vi "Test Basic Forms.vi"() -> ()   [LabVIEW 2020]
uses:
  lv-http-server/HTTP Server/Server/Server.lvclass
  lv-http-server/HTTP Server/RequestTraceLog/RequestTraceLog.lvclass
  lv-http-server/HTTP Server/StandardFileServe/StandardFileServe.lvclass
  lv-http-server/HTTP Server/Processing Step.ctl
  lv-http-server/HTTP Server/HTTP Server.lvlib
  lv-http-server/HTTP Server/Trace Item.ctl
  lv-http-server/HTTP Server/Trace Log.ctl
  lv-http-util/HTTP Utils/Method.ctl
  lv-http-util/HTTP Utils/HTTP Utils.lvlib
panel:
  in  "Debug":bool=TRUE
  out "error out":errorcluster
  in  "Port":u16=36987
  in  "Refresh Traces":bool
  out "Traces":T1[](array[typedef]) {"Sending" format="%_6f"; "Expires" format="%<%X %x>T"; "Created" format="%<%X %x>T"; "Waiting" format="%_6f"; "Parsing" format="%_6f"; "Processing" format="%_6f"; "Items"."Time" format="%.6f"; "Items"."Duration" format="%.6f"}
  # "Request"
  # "Response"
  # "Session"
  # "Auth"
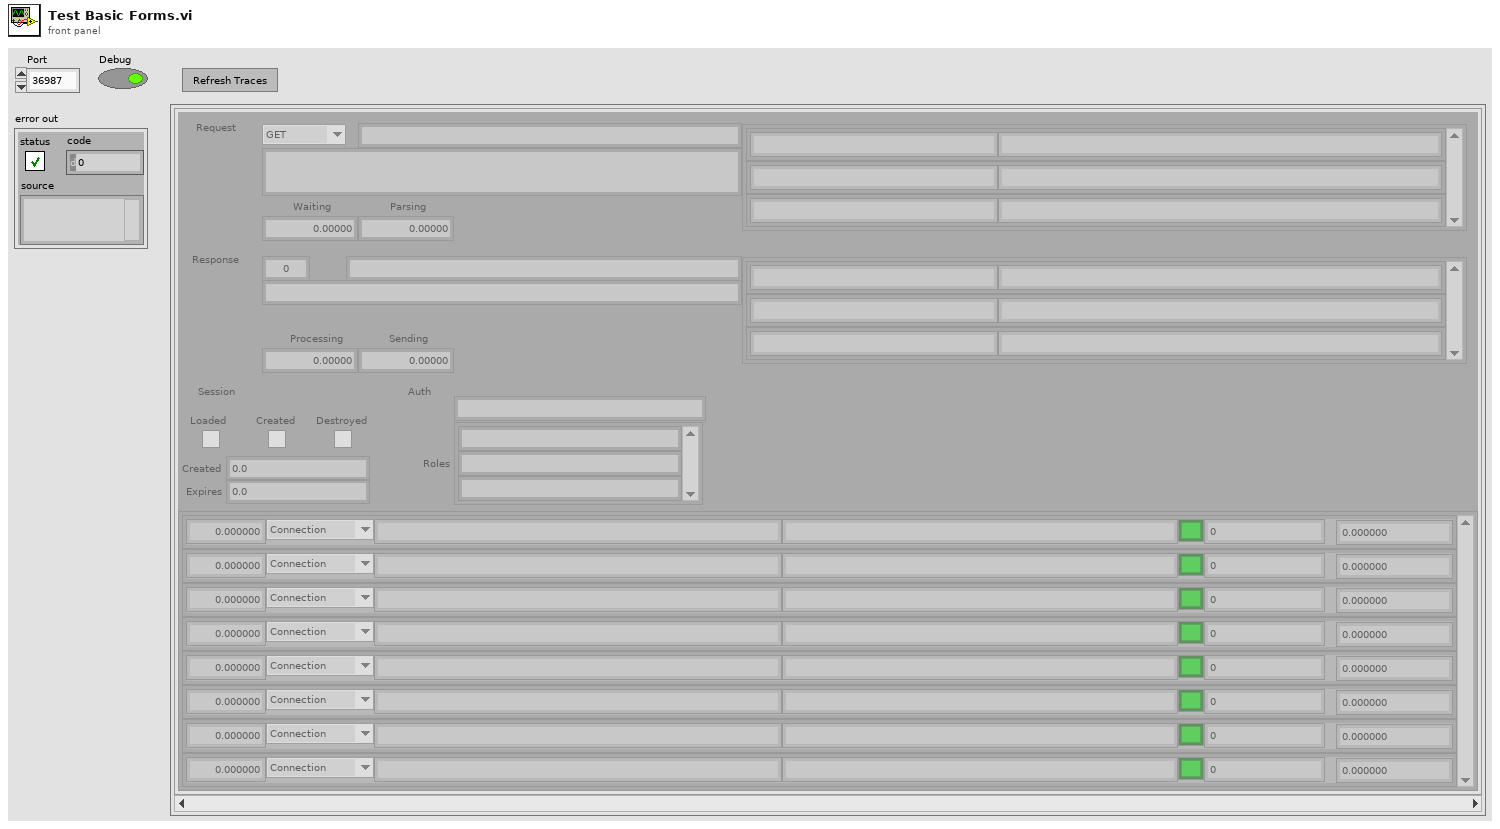
[diagram p1: front panel]
types:
  T1 = typedef "HTTP Server.lvlib/Trace Log.ctl" = cluster{"Items":T2[], "Client":string, "Target":string, "Response Type":string, "Processing":dbl, "Status":u16, "Method":T4, "Content Type":string, "Request Headers":cluster{"Name":string, "Value":string}[], "Parsing":dbl, "Waiting":dbl, "Identity":string, "Loaded":bool, "Created":bool, "Destroyed":bool, "Response Headers":cluster{"Name":string, "Value":string}[], "Created":dbl, "Expires":dbl, "Roles":string[], "Sending":dbl}
  T2 = typedef "HTTP Server.lvlib/Trace Item.ctl" = cluster{"Duration":dbl, "Step":T3, "Class":string, "Info":string, "Status":bool, "Code":i32, "Time":dbl}
  T3 = typedef "HTTP Server.lvlib/Processing Step.ctl" = enum16{"Connection", "Request", "Routing", "Controller Init", "Controller", "Response", "Complete", "Exception"}
  T4 = typedef "HTTP Utils.lvlib/Method.ctl" = enum16{"GET", "HEAD", "POST", "PUT", "DELETE", "CONNECT", "OPTIONS", "TRACE", "PATCH"}
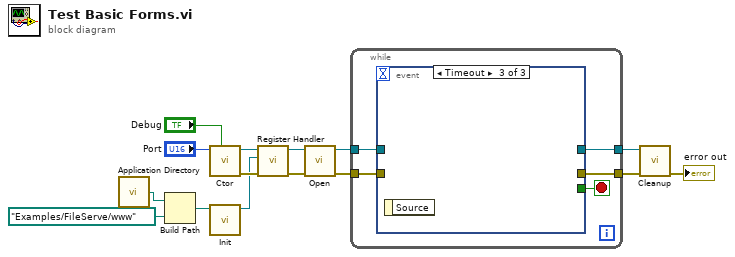
[diagram p0: block diagram]
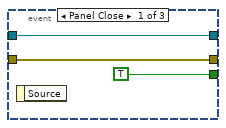
[diagram p2: hidden frame]
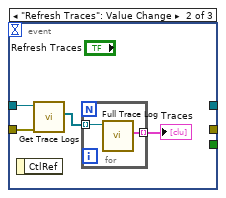
[diagram p3: hidden frame]
diagram:
  n1 = call <vilib>:"Application Directory.vi"() -> ("Application Directory"=w9:path)
  n2 = Build Path(base path=w9, name or relative path=path "Examples/FileServe/www") -> (appended path=w7:path)
  n3 = call "Ctor.vi"("Debug (F)"="Debug", "HTTP Port (80)"="Port") -> ("error out"=w3:errorcluster, "Server out"=w5:refnum<class "Server.lvclass">)  [unwired: 8 in]
  n4 = call "Init.vi"("Public Root"=w7) -> ("StandardFileServe out"=w1:refnum<class "StandardFileServe.lvclass">)  [unwired: 9 in, 1 out]
  n5 = call "Register Handler.vi"("error in (no error)"=w3, "Handler"=w1, "Server in"=w5) -> ("error out"=w2:errorcluster, "Server out"=w4:refnum<class "Server.lvclass">)  [unwired: 7 in]
  n6 = call "Open.vi"("error in (no error)"=w2, "Server in"=w4) -> ("error out"=w13:errorcluster, "Server out"=w14:refnum<class "Server.lvclass">)  [unwired: 8 in]
  n7 = while {
    tunnel: w14 -> [w18]
    tunnel: w13 -> [w19]
    tunnel: [w17] -> w12
    tunnel: [w16] -> w11
    stop <- w20 stop-if-true
    n8 = event shown="[2] Timeout" {
      selector: _ -> [_ _ _]
      dyn-events: _ -> [_ _ _]
      timeout: _ -> [_ _ _]
      tunnel: [TRUE ("Discard?") _ _] -> w20
      tunnel: w19 -> [w21 w26 _]
      tunnel: w18 -> [w22 w27 _]
      tunnel: [w22 _ _] -> w17
      tunnel: [w21 _ _] -> w16
      event Panel Close {
        n9 = event-data() -> ()  [unwired: 1 in, 1 out]
      }
      event "Refresh Traces": Value Change {
        n10 = event-data() -> ()  [unwired: 1 in, 1 out]
        n11 = call "Get Trace Logs.vi"("error in (no error)"=w26, "Server in"=w27) -> ("Trace Logs"=w25:refnum<class "RequestTraceLog.lvclass">[])  [unwired: 7 in, 2 out]
        n12 = for {
          tunnel: w25 -> [w29] mode=indexing
          tunnel: [w28] -> w24 mode=indexing
          n13 = call "Full Trace Log.vi"("RequestTraceLog in"=w29) -> ("Trace Log"=w28:T1)  [unwired: 8 in, 2 out]
        }
        "Traces" <- w24
      }
      event Timeout {
        n14 = event-data() -> ()  [unwired: 1 in, 1 out]
      }
    }
  }
  n15 = call "Cleanup.vi"("error in (no error)"=w11, "Server in"=w12) -> ("error out"=→"error out":errorcluster)  [unwired: 9 in]
